vi "Fifth Ex.vi"() -> ()   [LabVIEW 2016]
panel:
  in  "stop":bool
  out "Loops 3":i32
  out "Loops 2":i32
  out "Loops 1":i32
  out "Slide 4":dbl(slide) scale=0.0..10.0
  out "Slide 3":dbl(slide) scale=0.0..10.0
  out "Slide 2":dbl(slide) scale=0.0..10.0
  in  "Knob 3":dbl(knob) scale=0.0..10.0
  in  "Knob 2":dbl(knob) scale=0.0..10.0
  in  "Knob":dbl(knob) scale=0.0..10.0
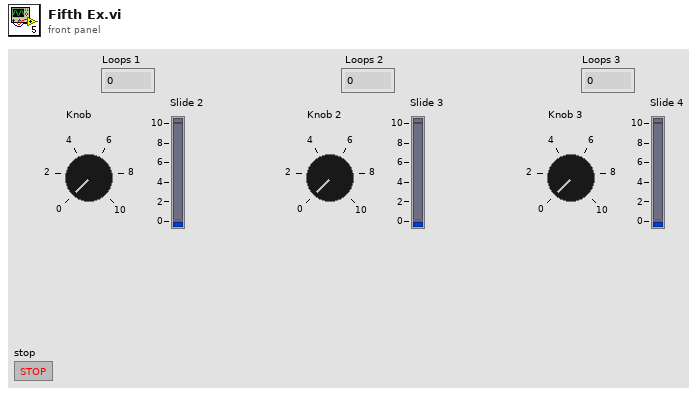
[diagram p1: front panel]
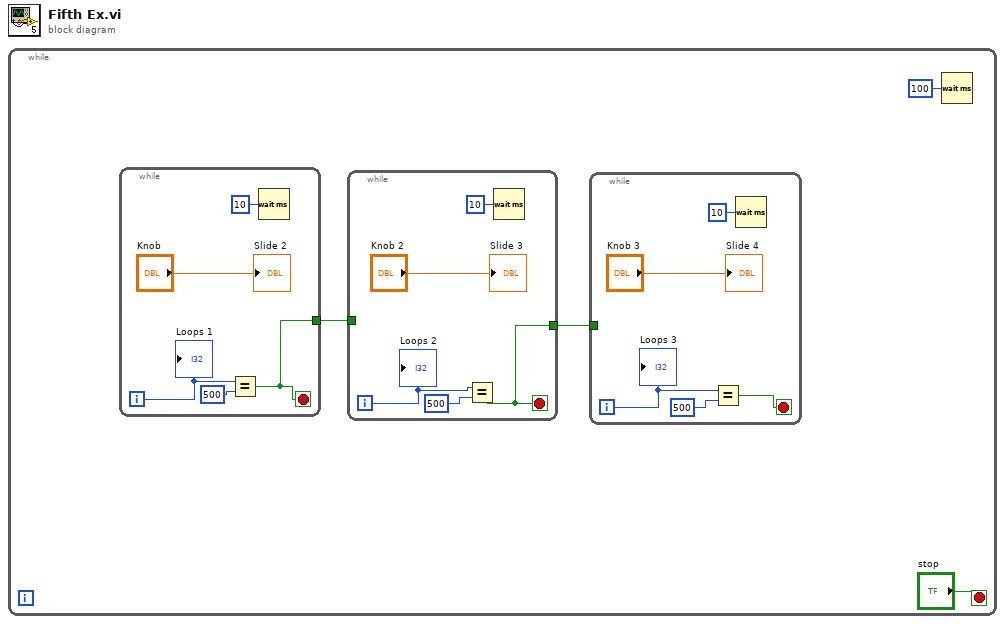
[diagram p0: block diagram]
diagram:
  n1 = while {
    stop <- "stop" stop-if-true
    n2 = while {
      tunnel: [w15] -> w4
      i -> [w17]
      stop <- w15 stop-if-true
      n3 = Equal?(x=w17, y=500) -> (x = y?=w15:bool)
      n4 = Wait (ms)(milliseconds to wait=u32 10) -> ()  [unwired: 1 out]
      "Slide 2" <- "Knob"
      "Loops 1" <- w17
    }
    n5 = while {
      tunnel: w4 -> [_]
      tunnel: [w10] -> w3
      i -> [w12]
      stop <- w10 stop-if-true
      n6 = Equal?(x=w12, y=500) -> (x = y?=w10:bool)
      n7 = Wait (ms)(milliseconds to wait=u32 10) -> ()  [unwired: 1 out]
      "Slide 3" <- "Knob 2"
      "Loops 2" <- w12
    }
    n8 = while {
      tunnel: w3 -> [_]
      i -> [w6]
      stop <- w7 stop-if-true
      n9 = Equal?(x=w6, y=500) -> (x = y?=w7:bool)
      n10 = Wait (ms)(milliseconds to wait=u32 10) -> ()  [unwired: 1 out]
      "Slide 4" <- "Knob 3"
      "Loops 3" <- w6
    }
    n11 = Wait (ms)(milliseconds to wait=u32 100) -> ()  [unwired: 1 out]
  }
